vi "5_6.vi"() -> ()   [LabVIEW 2015]
panel:
  out "Array":cluster{"XY Graph":cluster{dbl[], dbl[]}}[](array[cluster])
  in  "h":dbl
  in  "k":dbl
  in  "b":dbl
  in  "a":dbl
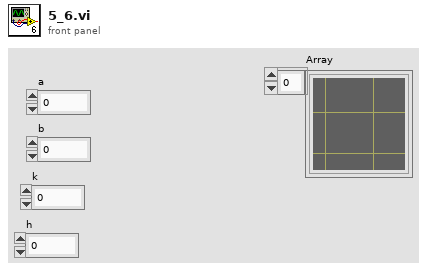
[diagram p1: front panel]
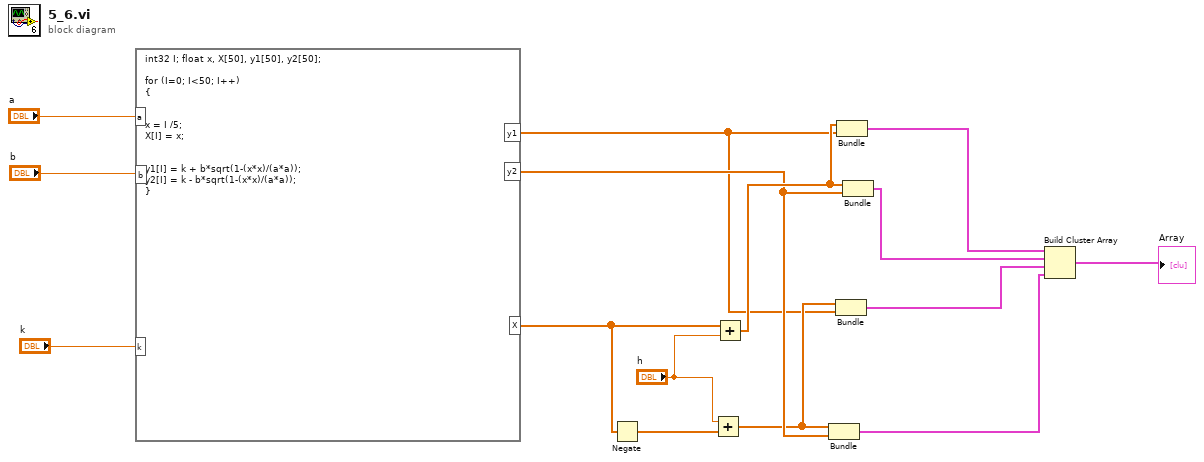
[diagram p0: block diagram]
diagram:
  n1 = formula code="int32 I; float x, X[50], y1[50], y2[50];\n\nfor (I=0; I<50; I++)\n{\n\n\nx = I /5;\nX[I] = x;\n\n\ny1[I] = k + b*sqrt(1-(x*x)/(a*a)); \ny2[I] = k - b*sqrt(1-(x*x)/(a*a)); \n}"("a"="a", "b"="b", "k"="k") -> ("y1"=w6:dbl[], "y2"=w8:dbl[], "X"=w12:dbl[])
  n2 = Negate(x=w12) -> (-x=w11:dbl[])
  n3 = Add(x="h", y=w11) -> (x+y=w7:dbl[])
  n4 = Add(x=w12, y="h") -> (x+y=w9:dbl[])
  n5 = Bundle(w7, w8) -> (w2:cluster{dbl[], dbl[]})  [unwired: 1 in]
  n6 = Bundle(w7, w6) -> (w3:cluster{dbl[], dbl[]})  [unwired: 1 in]
  n7 = Bundle(w9, w6) -> (w5:cluster{dbl[], dbl[]})  [unwired: 1 in]
  n8 = Bundle(w9, w8) -> (w4:cluster{dbl[], dbl[]})  [unwired: 1 in]
  n9 = Build Cluster Array(w5, w4, w3, w2) -> (→"Array":cluster{cluster{dbl[], dbl[]}}[])
